vi "VI Test.vi"   [LabVIEW 2016]
uses:
  Library/Classes/Pointer/Memory.Pointer.lvclass
  Library/Classes/Array/Memory.Array.lvclass
  Library/Classes/Pointer/Methods/Memory.Pointer.Write Bytes.Safe.vi
  Library/Classes/Pointer/Methods/Memory.Pointer.Read Bytes.Subset.In Place.Safe.vi
  Library/Classes/Pointer/Methods/Memory.Pointer.Read Bytes.Subset.Safe.vi
  Library/Classes/Pointer/Methods/Memory.Pointer.Move Block.Safe.vi
  Library/Classes/Pointer/Methods/Memory.Pointer.Offset to Address.Safe.vi
  Library/Classes/Pointer.DBL/Memory.Pointer.DBL.lvclass
  Library/Classes/Pointer.U64/Memory.Pointer.U64.lvclass
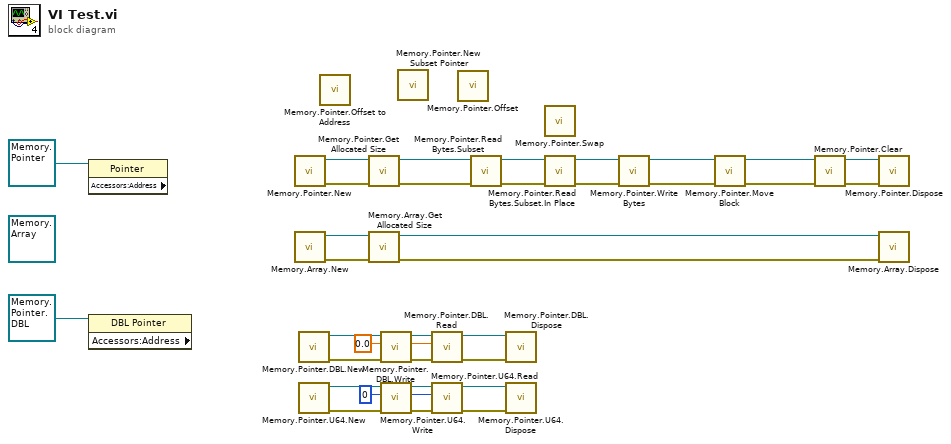
[diagram p0: block diagram]
diagram:
  (unwired) refnum<class "Memory.Array.lvclass"> refnum ("LabVIEW Memory Manager.lvlib:Array")
  n1 = property class="Pointer" props=["Accessors:Address"](reference=refnum<class "Memory.Pointer.lvclass"> refnum ("LabVIEW Memory Manager.lvlib:Pointer")) -> ()  [unwired: 1 in, 3 out]
  n2 = property class="DBL Pointer" props=["Accessors:Address"](reference=refnum<class "Memory.Pointer.DBL.lvclass"> refnum ("LabVIEW Memory Manager.lvlib:Memory.Pointer.DBL.lvclass")) -> ()  [unwired: 1 in, 3 out]
  n3 = call "Memory.Pointer.New.vi"() -> ("error out"=w32:errorcluster, "Pointer out"=w34:refnum<class "Memory.Pointer.lvclass">)  [unwired: 9 in, 1 out]
  n4 = call "Memory.Array.New.vi"() -> ("error out"=w33:errorcluster, "Array out"=w19:refnum<class "Memory.Array.lvclass">)  [unwired: 10 in]
  n5 = call "Memory.Pointer.DBL.New.vi"() -> ("error out"=w13:errorcluster, "DBL Pointer"=w16:refnum<class "Memory.Pointer.DBL.lvclass">)  [unwired: 10 in]
  n6 = call "Memory.Pointer.U64.New.vi"() -> ("error out"=w3:errorcluster, "U64 Pointer"=w4:refnum<class "Memory.Pointer.U64.lvclass">)  [unwired: 10 in]
  n7 = call-poly "Memory.Pointer.Offset to Address.vi"() -> ()  [unwired: 9 in, 3 out]
  n8 = call "Memory.Pointer.Get Allocated Size.vi"("error in (no error)"=w32, "Pointer in"=w34) -> ("error out"=w30:errorcluster, "Pointer out"=w18:refnum<class "Memory.Pointer.lvclass">)  [unwired: 7 in, 1 out]
  n9 = call "Memory.Array.Get Allocated Size.vi"("error in (no error)"=w33, "Array in"=w19) -> ("error out"=w24:errorcluster, "Array out"=w25:refnum<class "Memory.Array.lvclass">)  [unwired: 7 in, 1 out]
  n10 = call "Memory.Pointer.DBL.Write.vi"("error in (no error)"=w13, "value"=0.0, "DBL Pointer in"=w16) -> ("error out"=w12:errorcluster, "value out"=w10:dbl, "DBL Pointer out"=w15:refnum<class "Memory.Pointer.DBL.lvclass">)  [unwired: 6 in]
  n11 = call "Memory.Pointer.U64.Write.vi"("error in (no error)"=w3, "value"=u64 0, "U64 Pointer in"=w4) -> ("error out"=w7:errorcluster, "value out"=w9:u64, "U64 Pointer out"=w8:refnum<class "Memory.Pointer.U64.lvclass">)  [unwired: 6 in]
  n12 = call "Memory.Pointer.New Subset Pointer.vi"() -> ()  [unwired: 9 in, 3 out]
  n13 = call "Memory.Pointer.DBL.Read.vi"("error in (no error)"=w12, "value"=w10, "DBL Pointer in"=w15) -> ("error out"=w11:errorcluster, "DBL Pointer out"=w14:refnum<class "Memory.Pointer.DBL.lvclass">)  [unwired: 6 in, 1 out]
  n14 = call "Memory.Pointer.U64.Read.vi"("error in (no error)"=w7, "value"=w9, "U64 Pointer in"=w8) -> ("error out"=w5:errorcluster, "U64 Pointer out"=w6:refnum<class "Memory.Pointer.U64.lvclass">)  [unwired: 6 in, 1 out]
  n15 = call "Memory.Pointer.Offset.vi"() -> ()  [unwired: 10 in, 2 out]
  n16 = call-poly "Memory.Pointer.Read Bytes.Subset.vi"("error in (no error)"=w30, "Pointer in"=w18) -> ("error out"=w28:errorcluster, "Pointer out"=w29:refnum<class "Memory.Pointer.lvclass">)  [unwired: 6 in, 2 out]
  n17 = call "Memory.Pointer.DBL.Dispose.vi"("error in (no error)"=w11, "DBL Pointer"=w14) -> ()  [unwired: 9 in, 1 out]
  n18 = call "Memory.Pointer.U64.Dispose.vi"("error in (no error)"=w5, "U64 Pointer"=w6) -> ()  [unwired: 9 in, 1 out]
  n19 = call "Memory.Pointer.Swap.vi"() -> ()  [unwired: 9 in, 3 out]
  n20 = call-poly "Memory.Pointer.Read Bytes.Subset.In Place.vi"("error in (no error)"=w28, "Pointer in"=w29) -> ("error out"=w26:errorcluster, "Pointer out"=w27:refnum<class "Memory.Pointer.lvclass">)  [unwired: 6 in, 2 out]
  n21 = call-poly "Memory.Pointer.Write Bytes.vi"("error in (no error)"=w26, "Pointer in"=w27) -> ("error out"=w21:errorcluster, "Pointer out"=w23:refnum<class "Memory.Pointer.lvclass">)  [unwired: 6 in, 2 out]
  n22 = call-poly "Memory.Pointer.Move Block.vi"("src Pointer in"=w23, "error in (no error)"=w21) -> ("src Pointer out"=w22:refnum<class "Memory.Pointer.lvclass">, "error out"=w20:errorcluster)  [unwired: 11 in, 1 out]
  n23 = call "Memory.Pointer.Clear.vi"("error in (no error)"=w20, "Pointer in"=w22) -> ("error out"=w35:errorcluster, "Pointer out"=w36:refnum<class "Memory.Pointer.lvclass">)  [unwired: 8 in]
  n24 = call "Memory.Pointer.Dispose.vi"("error in (no error)"=w35, "Pointer in"=w36) -> ()  [unwired: 9 in, 1 out]
  n25 = call "Memory.Array.Dispose.vi"("error in (no error)"=w24, "Array in"=w25) -> ()  [unwired: 9 in, 1 out]
